vi "Validate Table Display Name.vi"(8 "error in":errorcluster, 11 "Table Display Name in":string) -> (0 "error out":errorcluster, 3 "Table Display Name out":string)   [LabVIEW 2019, in "Open Xml.lvlib"]
uses:
  Open Xml.lvlib
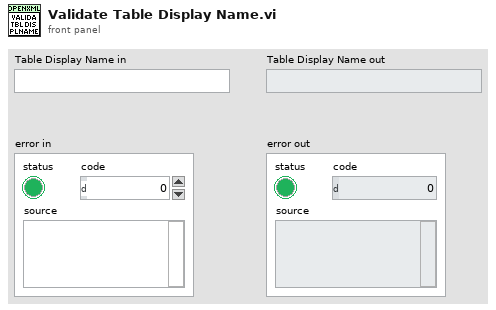
[diagram p1: front panel]
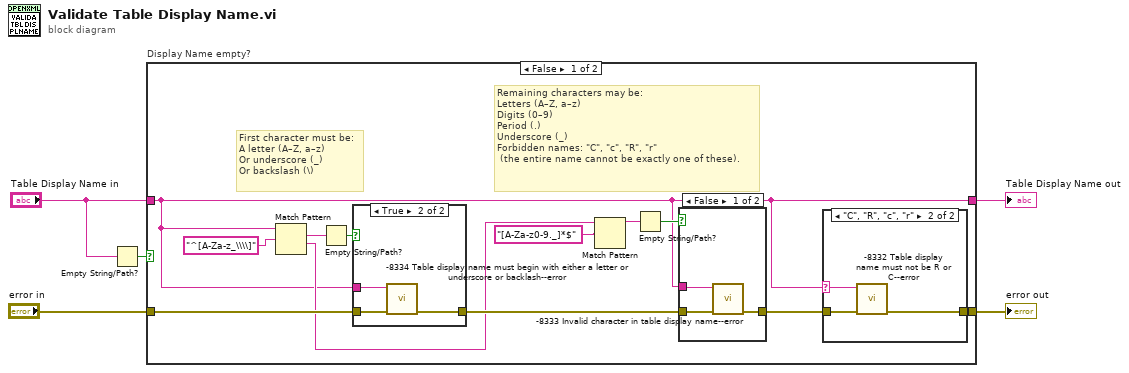
[diagram p0: block diagram]
diagram:
  n1 = Empty String/Path?(string/path="Table Display Name in") -> (empty?=w3:bool)
  n2 = case "Display Name empty?" shown="False" w3 {
    tunnel: "error in" -> [w17 w30]
    tunnel: [w8 w30] -> w4
    tunnel: "Table Display Name in" -> [w6 w31]
    tunnel: [w6 w31] -> w1
    frame False {
      # "Remaining characters may be:\nLetters (A–Z, a–z)\nDigits (0–9)\nPeriod (.)\nUnderscore (_)\nForbidden names: \"C\", \"c\", \"R\", \"r\"\n (the entire name cannot be exactly one of these)."
      # "First character must be:\nA letter (A–Z, a–z)\nOr underscore (_)\nOr backslash (\\)"
      n3 = Match Pattern(string=w6, regular expression="^[A-Za-z_\\\\]") -> (match substring=w14:string, after substring=w12:string)  [unwired: 1 in, 2 out]
      n4 = Empty String/Path?(string/path=w14) -> (empty?=w13:bool)
      n5 = case shown="True" w13 {
        tunnel: w17 -> [w26 w29]
        tunnel: [w26 w28] -> w16
        tunnel: w6 -> [_ w27]
        frame False {
        }
        frame True {
          n6 = call "-8334 Table display name must begin with either a letter or underscore or backlash--error.vi"("error in"=w29, "Argument"=w27) -> ("error out"=w28:errorcluster)  [unwired: 8 in, 1 out]
        }
      }
      n7 = Match Pattern(string=w12, regular expression="[A-Za-z0-9._]*$") -> (before substring=w7:string)  [unwired: 1 in, 3 out]
      n8 = Empty String/Path?(string/path=w7) -> (empty?=w11:bool)
      n9 = case shown="False" w11 {
        tunnel: w16 -> [w24 w25]
        tunnel: [w23 w25] -> w9
        tunnel: w6 -> [w22 _]
        frame False {
          n10 = call "-8333 Invalid character in table display name--error.vi"("error in"=w24, "Argument"=w22) -> ("error out"=w23:errorcluster)  [unwired: 8 in, 1 out]
        }
        frame True {
        }
      }
      n11 = case shown="\"C\", \"R\", \"c\", \"r\"" w6 {
        selector: w6 -> [_ w19]
        tunnel: w9 -> [w18 w21]
        tunnel: [w18 w20] -> w8
        frame "False", Default {
        }
        frame "C", "R", "c", "r" {
          n12 = call "-8332 Table display name must not be R or C--error.vi"("error in"=w21, "Argument"=w19) -> ("error out"=w20:errorcluster)  [unwired: 8 in, 1 out]
        }
      }
    }
    frame True {
    }
  }
  "error out" <- w4
  "Table Display Name out" <- w1
